vi "MultiSegmentSpectroscopy.vi"() -> ()   [LabVIEW 2019]
doc: "Performs a Bias Spectroscopy consisting of several user-definable segments.\n\n- Nanonis Programming Interface -"
uses:
  <userlib>/Nanonis Prog Interface V5/Nanonis Prog Interface.lvlib
panel:
  in  "Switch off Delay (s)":sgl min=0 max=100 format="%#_6p"
  in  "TipLift (m)":dbl format="%#_6p"
  out "SaveData":refnum<k4>
  in  "Save Data":bool
  out "Data":sgl[][](array[numeric])
  out "Index":u32[](array[numeric])
  out "UpdateGraphs":refnum<k4>
  out "RunSpec":refnum<k4>
  out "Change Params":refnum<k4>
  out "Sig_vs_Bias":cluster{sgl[], sgl[]}(graph)
  in  "Channel":u16(ring)
  out "Sig_vs_Ind":cluster{u32[], sgl[]}(graph)
  in  "Run Spectroscopy":bool
  out "Voltage Sequence":T1(graph)=[{"Data Points"=[0.0, 1.0, 2.0, 3.0, 4.0, 5.0, 6.0, 7.0, 8.0, 9.0, 10.0, 11.0, 12.0, 13.0, 14.0, 15.0, 16.0, 17.0, 18.0, 19.0, 20.0, 21.0, 22.0, 23.0, 24.0, 25.0, 26.0, 27.0, 28.0, 29.0, 30.0, 31.0, 32.0, 33.0, 34.0, 35.0, 36.0, 37.0, 38.0, 39.0, 40.0, 41.0, 42.0, 43.0, 44.0, 45.0, 46.0, 47.0, 48.0, 49.0], "Data Points"=[-1.0, -0.9836734693877551, -0.9673469387755103, -0.9510204081632653, -0.9346938775510204, -0.9183673469387755, -0.9020408163265305, -0.8857142857142857, -0.8693877551020408, -0.8530612244897959, -0.8367346938775511, -0.8204081632653061, -0.8040816326530612, -0.7877551020408163, -0.7714285714285714, -0.7551020408163265, -0.7387755102040816, -0.7224489795918367, -0.7061224489795919, -0.6897959183673469, -0.673469387755102, -0.6571428571428571, -0.6408163265306122, -0.6244897959183673, -0.6081632653061224, -0.5918367346938775, -0.5755102040816327, -0.5591836734693877, -0.5428571428571428, -0.5265306122448979, -0.510204081632653, -0.4938775510204081, -0.4775510204081632, -0.46122448979591835, -0.4448979591836735, -0.4285714285714285, -0.4122448979591836, -0.39591836734693875, -0.37959183673469377, -0.3632653061224489, -0.346938775510204, -0.33061224489795915, -0.3142857142857143, -0.2979591836734693, -0.2816326530612244, -0.26530612244897955, -0.24897959183673457, -0.2326530612244897, -0.21632653061224483, -0.19999999999999996]}, {"Data Points"=[50.0, 51.0, 52.0, 53.0, 54.0, 55.0, 56.0, 57.0, 58.0, 59.0, 60.0, 61.0, 62.0, 63.0, 64.0, 65.0, 66.0, 67.0, 68.0, 69.0, 70.0, 71.0, 72.0, 73.0, 74.0, 75.0, 76.0, 77.0, 78.0, 79.0, 80.0, 81.0, 82.0, 83.0, 84.0, 85.0, 86.0, 87.0, 88.0, 89.0, 90.0, 91.0, 92.0, 93.0, 94.0, 95.0, 96.0, 97.0, 98.0, 99.0, 100.0, 101.0, 102.0, 103.0, 104.0, 105.0, 106.0, 107.0, 108.0, 109.0, 110.0, 111.0, 112.0, 113.0, 114.0, 115.0, 116.0, 117.0, 118.0, 119.0, 120.0, 121.0, 122.0, 123.0, 124.0, 125.0, 126.0, 127.0, 128.0, 129.0, 130.0, 131.0, 132.0, 133.0, 134.0, 135.0, 136.0, 137.0, 138.0, 139.0, 140.0, 141.0, 142.0, 143.0, 144.0, 145.0, 146.0, 147.0, 148.0, 149.0, 150.0, 151.0, 152.0, 153.0, 154.0, 155.0, 156.0, 157.0, 158.0, 159.0, 160.0, 161.0, 162.0, 163.0, 164.0, 165.0, 166.0, 167.0, 168.0, 169.0, 170.0, 171.0, 172.0, 173.0, 174.0, 175.0, 176.0, 177.0, 178.0, 179.0, 180.0, 181.0, 182.0, 183.0, 184.0, 185.0, 186.0, 187.0, 188.0, 189.0, 190.0, 191.0, 192.0, 193.0, 194.0, 195.0, 196.0, 197.0, 198.0, 199.0, 200.0, 201.0, 202.0, 203.0, 204.0, 205.0, 206.0, 207.0, 208.0, 209.0, 210.0, 211.0, 212.0, 213.0, 214.0, 215.0, 216.0, 217.0, 218.0, 219.0, 220.0, 221.0, 222.0, 223.0, 224.0, 225.0, 226.0, 227.0, 228.0, 229.0, 230.0, 231.0, 232.0, 233.0, 234.0, 235.0, 236.0, 237.0, 238.0, 239.0, 240.0, 241.0, 242.0, 243.0, 244.0, 245.0, 246.0, 247.0, 248.0, 249.0, 250.0, 251.0, 252.0, 253.0, 254.0, 255.0, 256.0, 257.0, 258.0, 259.0, 260.0, 261.0, 262.0, 263.0, 264.0, 265.0, 266.0, 267.0, 268.0, 269.0, 270.0, 271.0, 272.0, 273.0, 274.0, 275.0, 276.0, 277.0, 278.0, 279.0, 280.0, 281.0, 282.0, 283.0, 284.0, 285.0, 286.0, 287.0, 288.0, 289.0, 290.0, 291.0, 292.0, 293.0, 294.0, 295.0, 296.0, 297.0, 298.0, 299.0, 300.0, 301.0, 302.0, 303.0, 304.0, 305.0, 306.0, 307.0, 308.0, 309.0, 310.0, 311.0, 312.0, 313.0, 314.0, 315.0, 316.0, 317.0, 318.0, 319.0, 320.0, 321.0, 322.0, 323.0, 324.0, 325.0, 326.0, 327.0, 328.0, 329.0, 330.0, 331.0, 332.0, 333.0, 334.0, 335.0, 336.0, 337.0, 338.0, 339.0, 340.0, 341.0, 342.0, 343.0, 344.0, 345.0, 346.0, 347.0, 348.0, 349.0, 350.0, 351.0, 352.0, 353.0, 354.0, 355.0, 356.0, 357.0, 358.0, 359.0, 360.0, 361.0, 362.0, 363.0, 364.0, 365.0, 366.0, 367.0, 368.0, 369.0, 370.0, 371.0, 372.0, 373.0, 374.0, 375.0, 376.0, 377.0, 378.0, 379.0, 380.0, 381.0, 382.0, 383.0, 384.0, 385.0, 386.0, 387.0, 388.0, 389.0, 390.0, 391.0, 392.0, 393.0, 394.0, 395.0, 396.0, 397.0, 398.0, 399.0, 400.0, 401.0, 402.0, 403.0, 404.0, 405.0, 406.0, 407.0, 408.0, 409.0, 410.0, 411.0, 412.0, 413.0, 414.0, 415.0, 416.0, 417.0, 418.0, 419.0, 420.0, 421.0, 422.0, 423.0, 424.0, 425.0, 426.0, 427.0, 428.0, 429.0, 430.0, 431.0, 432.0, 433.0, 434.0, 435.0, 436.0, 437.0, 438.0, 439.0, 440.0, 441.0, 442.0, 443.0, 444.0, 445.0, 446.0, 447.0, 448.0, 449.0], "Data Points"=[-0.2, -0.19899749373433584, -0.1979949874686717, -0.19699248120300752, -0.19598997493734338, -0.1949874686716792, -0.19398496240601504, -0.1929824561403509, -0.19197994987468672, -0.19097744360902258, -0.1899749373433584, -0.18897243107769424, -0.1879699248120301, -0.18696741854636592, -0.18596491228070178, -0.1849624060150376, -0.18395989974937343, -0.1829573934837093, -0.18195488721804512, -0.18095238095238098, -0.1799498746867168, -0.17894736842105263, -0.1779448621553885, -0.17694235588972432, -0.17593984962406017, -0.174937343358396, -0.17393483709273183, -0.1729323308270677, -0.17192982456140352, -0.17092731829573937, -0.1699248120300752, -0.16892230576441103, -0.16791979949874689, -0.16691729323308271, -0.16591478696741857, -0.1649122807017544, -0.16390977443609023, -0.16290726817042608, -0.1619047619047619, -0.16090225563909777, -0.1598997493734336, -0.15889724310776943, -0.15789473684210528, -0.1568922305764411, -0.15588972431077697, -0.1548872180451128, -0.15388471177944862, -0.15288220551378448, -0.1518796992481203, -0.15087719298245617, -0.149874686716792, -0.14887218045112782, -0.14786967418546368, -0.1468671679197995, -0.14586466165413536, -0.1448621553884712, -0.14385964912280702, -0.14285714285714288, -0.1418546365914787, -0.14085213032581456, -0.1398496240601504, -0.13884711779448622, -0.13784461152882208, -0.1368421052631579, -0.13583959899749376, -0.1348370927318296, -0.13383458646616542, -0.13283208020050125, -0.1318295739348371, -0.13082706766917296, -0.1298245614035088, -0.12882205513784462, -0.12781954887218044, -0.1268170426065163, -0.12581453634085216, -0.12481203007518799, -0.12380952380952383, -0.12280701754385966, -0.1218045112781955, -0.12080200501253134, -0.11979949874686718, -0.11879699248120303, -0.11779448621553885, -0.1167919799498747, -0.11578947368421054, -0.11478696741854638, -0.11378446115288222, -0.11278195488721805, -0.1117794486215539, -0.11077694235588974, -0.10977443609022558, -0.10877192982456142, -0.10776942355889725, -0.1067669172932331, -0.10576441102756894, -0.10476190476190478, -0.1037593984962406, -0.10275689223057645, -0.10175438596491229, -0.10075187969924813, -0.09974937343358398, -0.0987468671679198, -0.09774436090225565, -0.09674185463659149, -0.09573934837092733, -0.09473684210526317, -0.093734335839599, -0.09273182957393485, -0.09172932330827069, -0.09072681704260653, -0.08972431077694237, -0.0887218045112782, -0.08771929824561404, -0.08671679197994989, -0.08571428571428573, -0.08471177944862157, -0.0837092731829574, -0.08270676691729324, -0.08170426065162908, -0.08070175438596493, -0.07969924812030077, -0.0786967418546366, -0.07769423558897244, -0.07669172932330828, -0.07568922305764413, -0.07468671679197997, -0.0736842105263158, -0.07268170426065165, -0.07167919799498748, -0.07067669172932331, -0.06967418546365917, -0.068671679197995, -0.06766917293233085, -0.06666666666666668, -0.06566416040100251, -0.06466165413533836, -0.06365914786967419, -0.06265664160401005, -0.06165413533834588, -0.060651629072681706, -0.05964912280701756, -0.05864661654135339, -0.05764411027568925, -0.056641604010025076, -0.055639097744360905, -0.05463659147869676, -0.05363408521303259, -0.052631578947368446, -0.051629072681704274, -0.0506265664160401, -0.04962406015037596, -0.04862155388471179, -0.047619047619047644, -0.04661654135338347, -0.0456140350877193, -0.04461152882205516, -0.043609022556390986, -0.04260651629072684, -0.04160401002506267, -0.0406015037593985, -0.039598997493734356, -0.038596491228070184, -0.03759398496240604, -0.03659147869674187, -0.0355889724310777, -0.034586466165413554, -0.03358395989974938, -0.03258145363408524, -0.03157894736842107, -0.030576441102756896, -0.029573934837092752, -0.02857142857142858, -0.027568922305764437, -0.026566416040100266, -0.025563909774436094, -0.02456140350877195, -0.02355889724310778, -0.022556390977443636, -0.021553884711779464, -0.020551378446115293, -0.01954887218045115, -0.018546365914786977, -0.017543859649122834, -0.016541353383458662, -0.015538847117794491, -0.014536340852130347, -0.013533834586466176, -0.012531328320802032, -0.01152882205513786, -0.01052631578947369, -0.009523809523809545, -0.008521303258145374, -0.007518796992481203, -0.006516290726817059, -0.0055137844611528875, -0.004511278195488744, -0.0035087719298245723, -0.002506265664160401, -0.0015037593984962572, -0.0005012531328320857, 0.000501253132832058, 0.0015037593984962294, 0.002506265664160401, 0.0035087719298245446, 0.004511278195488716, 0.00551378446115286, 0.006516290726817031, 0.007518796992481203, 0.008521303258145346, 0.009523809523809518, 0.010526315789473661, 0.011528822055137833, 0.012531328320802004, 0.013533834586466148, 0.01453634085213032, 0.015538847117794463, 0.016541353383458635, 0.017543859649122806, 0.01854636591478695, 0.01954887218045112, 0.020551378446115265, 0.021553884711779436, 0.022556390977443608, 0.02355889724310775, 0.024561403508771923, 0.025563909774436067, 0.026566416040100238, 0.02756892230576441, 0.028571428571428553, 0.029573934837092725, 0.03057644110275687, 0.03157894736842104, 0.03258145363408521, 0.033583959899749355, 0.034586466165413526, 0.03558897243107767, 0.03659147869674184, 0.03759398496240601, 0.03859649122807016, 0.03959899749373433, 0.04060150375939847, 0.04160401002506264, 0.042606516290726815, 0.04360902255639096, 0.04461152882205513, 0.045614035087719274, 0.046616541353383445, 0.047619047619047616, 0.04862155388471176, 0.04962406015037593, 0.050626566416040075, 0.05162907268170425, 0.05263157894736842, 0.05363408521303259, 0.054636591478696706, 0.05563909774436088, 0.05664160401002505, 0.05764411027568922, 0.05864661654135339, 0.05964912280701751, 0.06065162907268168, 0.06165413533834585, 0.06265664160401002, 0.06365914786967419, 0.06466165413533831, 0.06566416040100248, 0.06666666666666665, 0.06766917293233082, 0.068671679197995, 0.06967418546365911, 0.07067669172932328, 0.07167919799498745, 0.07268170426065163, 0.0736842105263158, 0.07468671679197991, 0.07568922305764408, 0.07669172932330826, 0.07769423558897243, 0.0786967418546366, 0.07969924812030071, 0.08070175438596489, 0.08170426065162906, 0.08270676691729323, 0.0837092731829574, 0.08471177944862152, 0.08571428571428569, 0.08671679197994986, 0.08771929824561403, 0.0887218045112782, 0.08972431077694232, 0.09072681704260649, 0.09172932330827066, 0.09273182957393483, 0.093734335839599, 0.09473684210526312, 0.09573934837092729, 0.09674185463659146, 0.09774436090225563, 0.0987468671679198, 0.09974937343358392, 0.10075187969924809, 0.10175438596491226, 0.10275689223057644, 0.1037593984962406, 0.10476190476190472, 0.1057644110275689, 0.10676691729323307, 0.10776942355889724, 0.10877192982456141, 0.10977443609022552, 0.1107769423558897, 0.11177944862155387, 0.11278195488721804, 0.11378446115288221, 0.11478696741854633, 0.1157894736842105, 0.11679197994987467, 0.11779448621553884, 0.11879699248120301, 0.11979949874686713, 0.1208020050125313, 0.12180451127819547, 0.12280701754385964, 0.12380952380952381, 0.12481203007518793, 0.1258145363408521, 0.12681704260651627, 0.12781954887218044, 0.12882205513784462, 0.12982456140350873, 0.1308270676691729, 0.13182957393483707, 0.13283208020050125, 0.13383458646616542, 0.13483709273182953, 0.1358395989974937, 0.13684210526315788, 0.13784461152882205, 0.13884711779448622, 0.13984962406015033, 0.1408521303258145, 0.14185463659147868, 0.14285714285714285, 0.14385964912280702, 0.14486215538847114, 0.1458646616541353, 0.14686716791979948, 0.14786967418546365, 0.14887218045112782, 0.14987468671679194, 0.1508771929824561, 0.15187969924812028, 0.15288220551378445, 0.15388471177944862, 0.15488721804511274, 0.1558897243107769, 0.15689223057644108, 0.15789473684210525, 0.15889724310776943, 0.15989974937343354, 0.1609022556390977, 0.16190476190476188, 0.16290726817042606, 0.16390977443609023, 0.16491228070175434, 0.16591478696741851, 0.1669172932330827, 0.16791979949874686, 0.16892230576441103, 0.16992481203007515, 0.17092731829573932, 0.1719298245614035, 0.17293233082706766, 0.17393483709273183, 0.17493734335839595, 0.17593984962406012, 0.1769423558897243, 0.17794486215538846, 0.17894736842105263, 0.17994987468671675, 0.18095238095238092, 0.1819548872180451, 0.18295739348370926, 0.18395989974937343, 0.1849624060150376, 0.18596491228070172, 0.1869674185463659, 0.18796992481203006, 0.18897243107769424, 0.1899749373433584, 0.19097744360902252, 0.1919799498746867, 0.19298245614035087, 0.19398496240601504, 0.1949874686716792, 0.19598997493734333, 0.1969924812030075, 0.19799498746867167, 0.19899749373433584, 0.2]}, ...(3 in all)]
  out "AllQuit":bool
  in  "stop":bool
  in  "Autosave Data":enum16{"no change", "on", "off"}(ring)
  in  "Parameters":T2(array[cluster])=[{"Start"=-1.0, "Stop"=-0.2, "# Points"=50}, {"Start"=-0.2, "Stop"=0.2, "# Points"=400}, {"Start"=0.2, "Stop"=1.0, "# Points"=50}] {"# Points" min=2; "Stop" format="%1_3p"; "Start" format="%1_3p"}
  # "Temporary Variables"
  # "Z-Controller"
  # "Note:\nTo insert or remove a \nsegment right-click in \nthe parameter section"
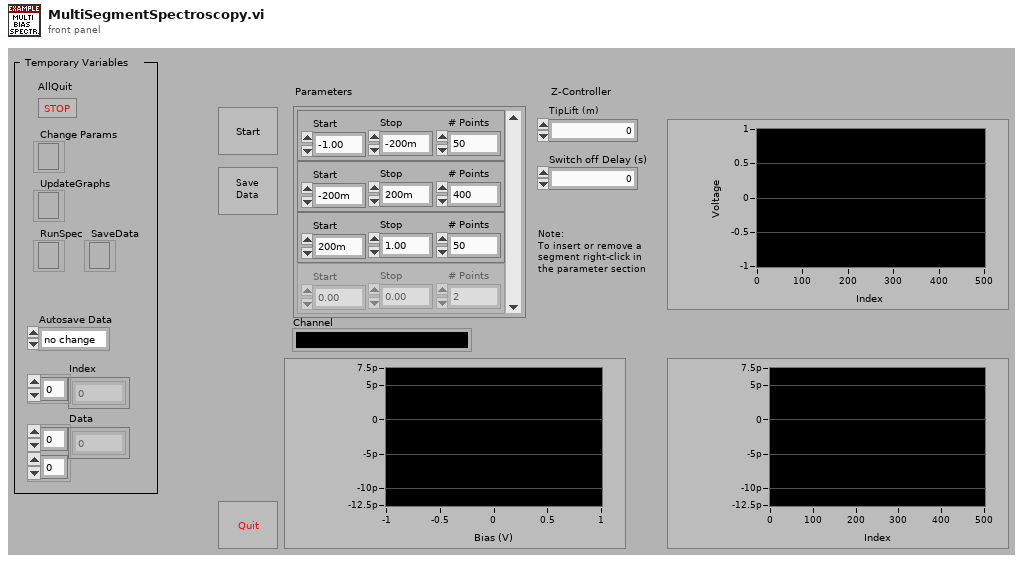
[diagram p1: front panel]
types:
  T1 = cluster{"Data Points":dbl[], "Data Points":dbl[]}[]
  T2 = cluster{"Start":dbl, "Stop":dbl, "# Points":i32}[]
  T3 = cluster{"Data Points":dbl[], "Data Points":dbl[]}
  T4 = cluster{"End settling time (s)":sgl, "Z control time (s)":sgl}
  T5 = cluster{"Z averaging time (s)":sgl, "Z offset (m)":sgl, "Initial settling time (s)":sgl}
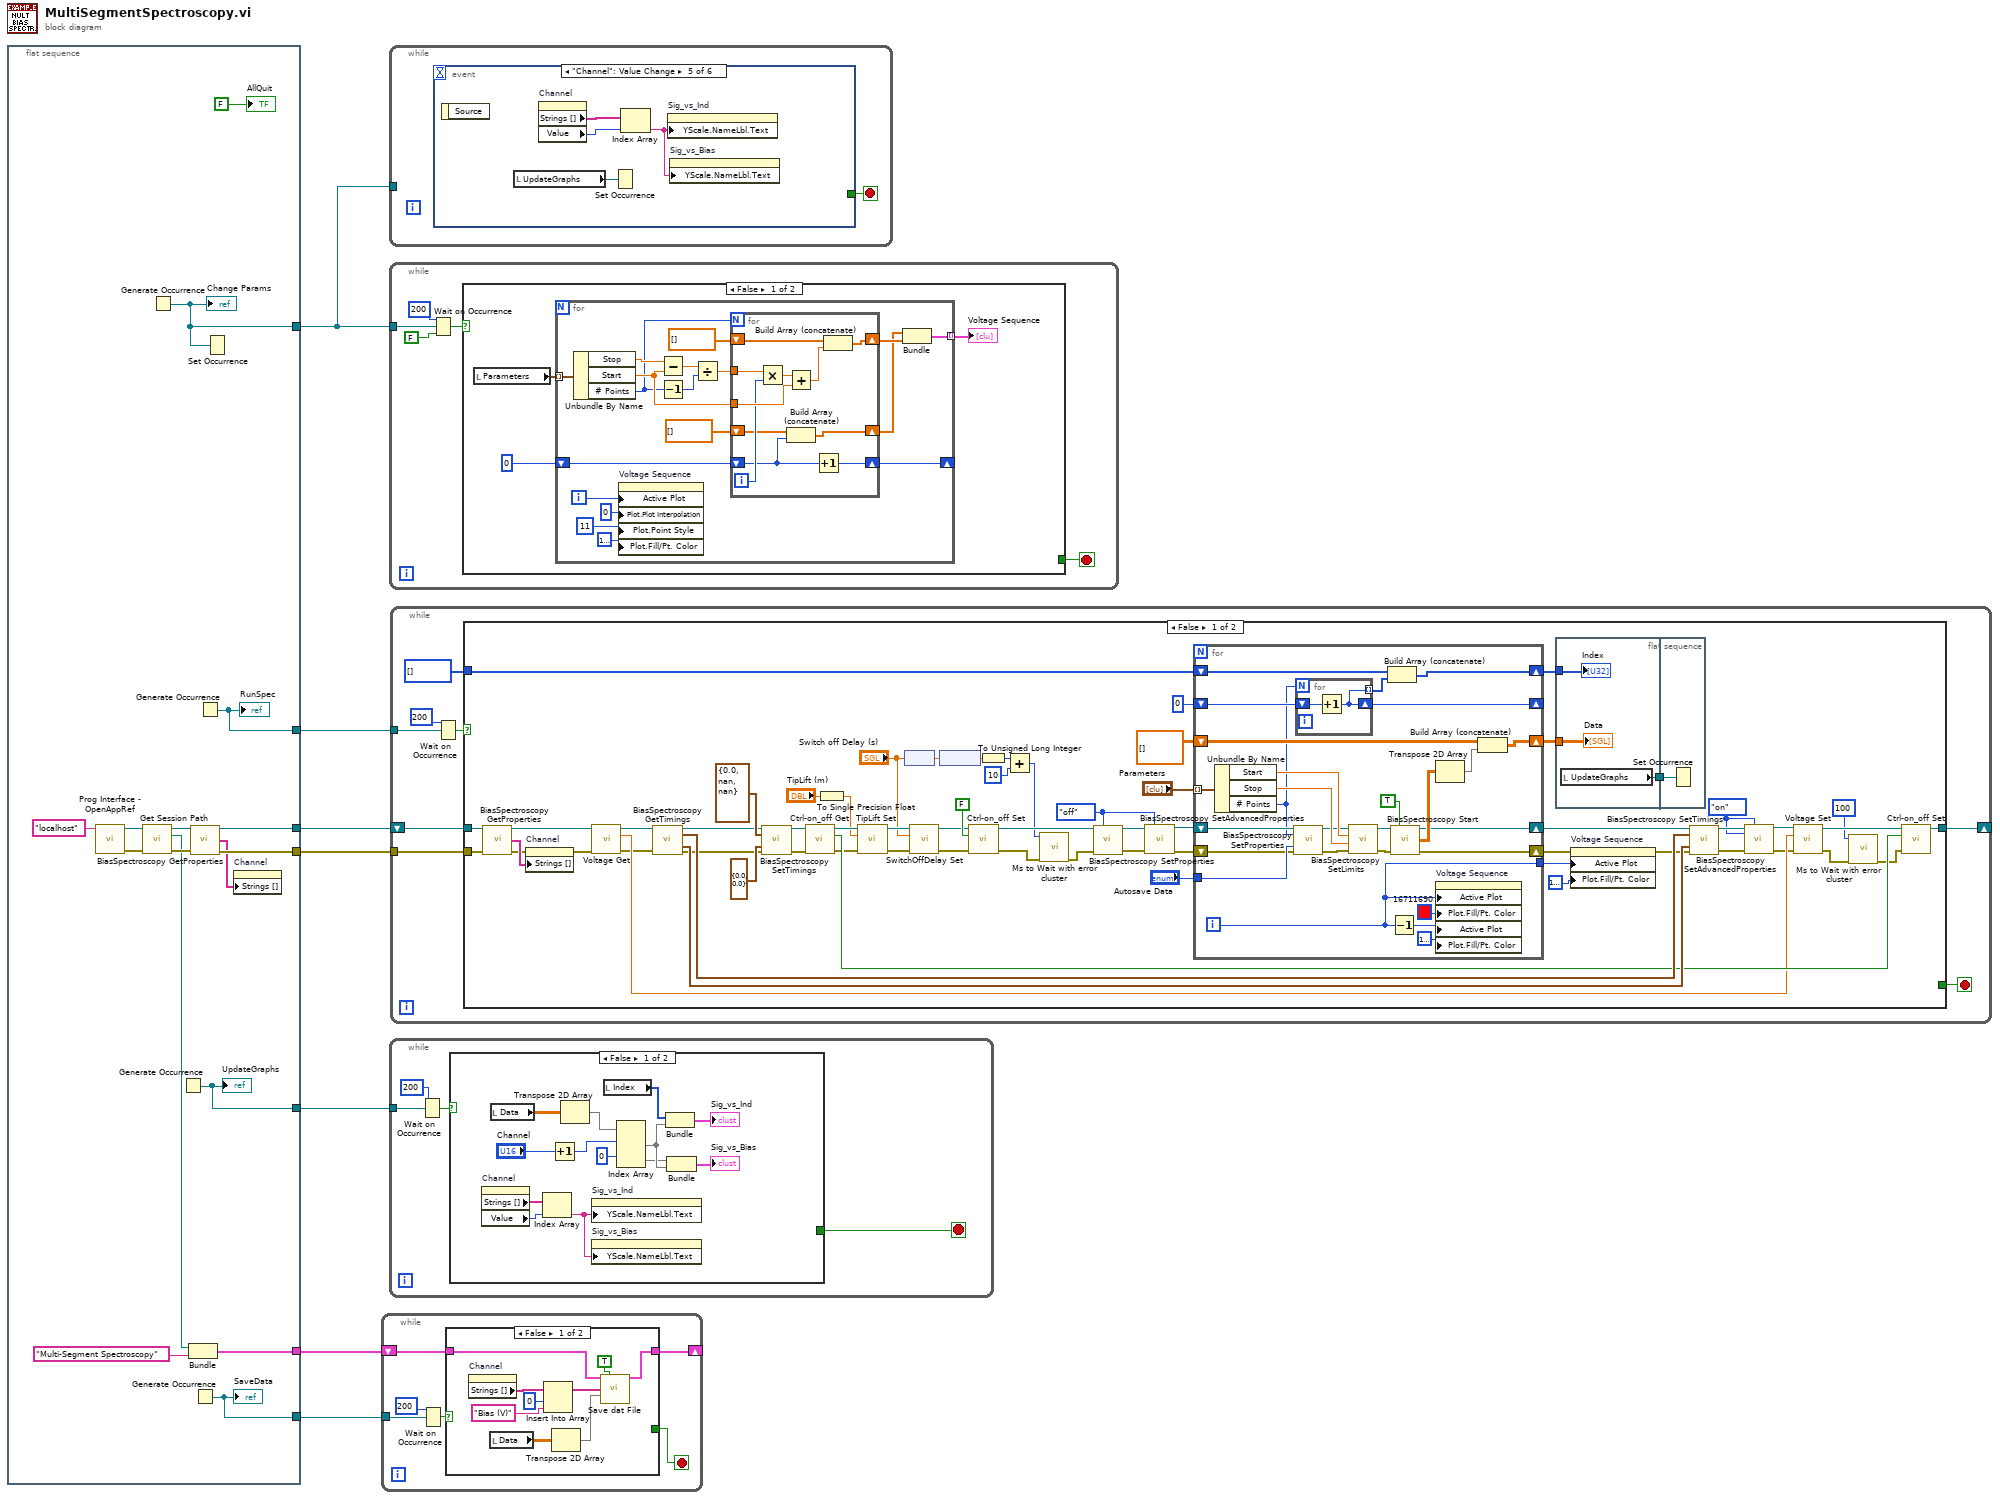
[diagram p0: block diagram]
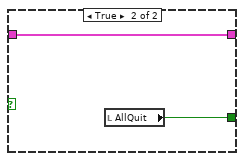
[diagram p2: hidden frame]
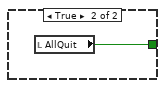
[diagram p3: hidden frame]
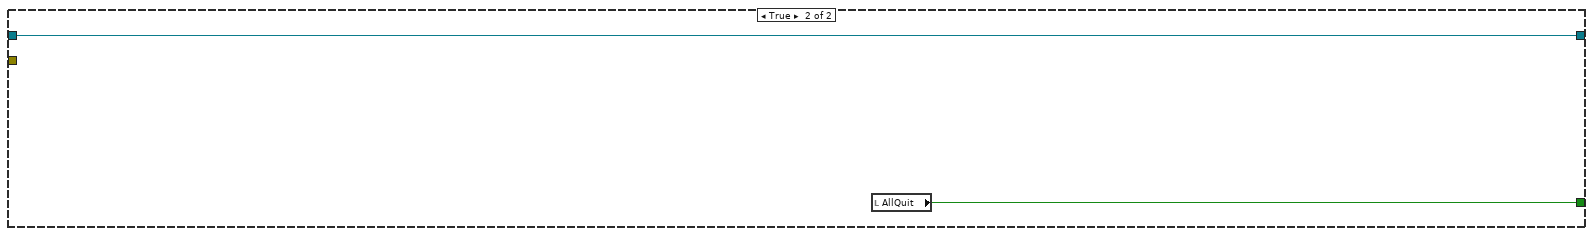
[diagram p4: hidden frame]
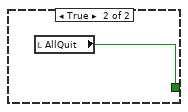
[diagram p5: hidden frame]
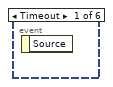
[diagram p6: hidden frame]
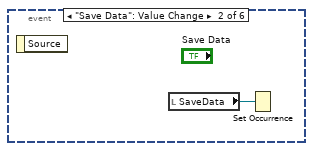
[diagram p7: hidden frame]
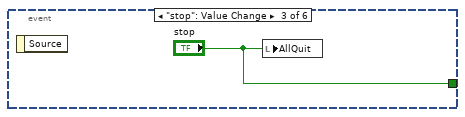
[diagram p8: hidden frame]
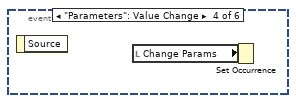
[diagram p9: hidden frame]
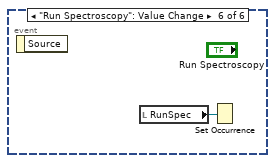
[diagram p10: hidden frame]
diagram:
  n1 = flat-sequence {
    tunnel: [w19] -> w7
    tunnel: [w20] -> w5
    tunnel: [w17] -> w6
    tunnel: [w21] -> w4
    tunnel: [w18] -> w3
    tunnel: [w16] -> w2
    tunnel: [w8] -> w1
    frame #0 {
      n2 = call <userlib>:"Prog Interface - OpenAppRef.vi"("Machine name (local machine IP)"="localhost" ("Machine name (localhost)")) -> ("Error out"=w11:errorcluster, "Application reference"=w14:refnum<vi>)  [unwired: 5 in]
      n3 = call <userlib>:"Get Session Path.vi"("error in (no error)"=w11, "Application ref in"=w14) -> ("error out"=w12:errorcluster, "Session path"=w9:path, "Application ref out"=w13:refnum<vi>)  [unwired: 7 in]
      n4 = Generate Occurrence() -> (w20:refnum<k4>)
      "Change Params" <- w20
      n5 = Generate Occurrence() -> (w21:refnum<k4>)
      "UpdateGraphs" <- w21
      n6 = Bundle("Session path"=w9, "Basename"="Multi-Segment Spectroscopy") -> (w8:cluster{"Session path":path, "Basename":string})  [unwired: 1 in]
      n7 = call <userlib>:"BiasSpectroscopy GetProperties.vi"("Application ref in"=w13, "Error in (no error)"=w12) -> ("Application ref out"=w16:refnum<vi>, "Channels"=w15:string[], "Error out"=w19:errorcluster)  [unwired: 6 in, 5 out]
      n8 = Generate Occurrence() -> (w18:refnum<k4>)
      "SaveData" <- w18
      n9 = Generate Occurrence() -> (w17:refnum<k4>)
      "RunSpec" <- w17
      n10 = Set Occurrence(w20) -> ()
      n11 = property on="Channel" class="Ring (strict)"("Strings []"=w15) -> ()  [unwired: 2 in, 2 out]
      "AllQuit" <- FALSE ("AllQuit")
    }
  }
  n12 = while {
    tunnel: w3 -> [w27]
    shift-right: [w24] -> _
    shift-left: w1 -> [w25]
    stop <- w28 stop-if-true
    n13 = Wait on Occurrence(2:w27, 3:200 ("ms timeout (-1)")) -> (0:w29:bool)  [unwired: 1 in]
    n14 = case shown="False" w29 {
      tunnel: [_ w40] -> w28
      tunnel: w25 -> [w31 w39]
      tunnel: [w30 w39] -> w24
      frame False {
        n15 = property on="Channel" class="Ring (strict)"() -> ("Strings []"=w37:string[])  [unwired: 2 in, 2 out]
        n16 = local read "Data"() -> (w34:sgl[][])
        n17 = Insert Into Array(array=w37, index=0, new element="Bias (V)") -> (w35:string[])
        n18 = Transpose 2D Array(2D array=w34) -> (transposed array=w33:sgl[][])
        n19 = call <userlib>:"Save dat File.vi"("Filename control"=w31, "Show save dialog (T)"=TRUE, "Channels names"=w35, "Data"=w33) -> ("Filename control out"=w30:cluster{"Path":path, "Basename":string})  [unwired: 8 in, 3 out]
      }
      frame True {
        n20 = local read "AllQuit"() -> (w40:bool)
      }
    }
  }
  n21 = while {
    tunnel: w5 -> [_]
    stop <- w41 stop-if-true
    n22 = event shown="[4] \"Channel\": Value Change" {
      selector: _ -> [_ _ _ _ _ _]
      dyn-events: _ -> [_ _ _ _ _ _]
      timeout: _ -> [_ _ _ _ _ _]
      tunnel: [_ _ "stop" _ _ _] -> w41
      event Timeout {
        n23 = event-data() -> ()  [unwired: 1 in, 1 out]
      }
      event "Save Data": Value Change {
        n24 = event-data() -> ()  [unwired: 1 in, 1 out]
        n25 = local read "SaveData"() -> (w42:refnum<k4>)
        n26 = Set Occurrence(w42) -> ()
      }
      event "stop": Value Change {
        n27 = event-data() -> ()  [unwired: 1 in, 1 out]
        n28 = local write "AllQuit"("stop") -> ()
      }
      event "Parameters": Value Change {
        n29 = event-data() -> ()  [unwired: 1 in, 1 out]
        n30 = local read "Change Params"() -> (w44:refnum<k4>)
        n31 = Set Occurrence(w44) -> ()
      }
      event "Channel": Value Change {
        n32 = event-data() -> ()  [unwired: 1 in, 1 out]
        n33 = local read "UpdateGraphs"() -> (w46:refnum<k4>)
        n34 = property on="Channel" class="Ring (strict)"() -> ("Strings []"=w48:string[], "Value"=w45:u16)  [unwired: 2 in, 2 out]
        n35 = Set Occurrence(w46) -> ()
        n36 = Index Array(array=w48, index=w45) -> (element=w47:string)
        n37 = property on="Sig_vs_Ind" class="XYGraph (strict)"("YScale.NameLbl.Text"=w47) -> ()  [unwired: 2 in, 2 out]
        n38 = property on="Sig_vs_Bias" class="XYGraph (strict)"("YScale.NameLbl.Text"=w47) -> ()  [unwired: 2 in, 2 out]
      }
      event "Run Spectroscopy": Value Change {
        n39 = event-data() -> ()  [unwired: 1 in, 1 out]
        n40 = local read "RunSpec"() -> (w49:refnum<k4>)
        n41 = Set Occurrence(w49) -> ()
      }
    }
  }
  n42 = while {
    tunnel: w5 -> [w54]
    stop <- w51 stop-if-true
    n43 = Wait on Occurrence(1:FALSE ("ignore previous (T)"), 2:w54, 3:200 ("ms timeout (-1)")) -> (0:w52:bool)
    n44 = case shown="False" w52 {
      tunnel: [_ w87] -> w51
      frame False {
        n45 = local read "Parameters"() -> (w55:T2)
        n46 = for {
          shift-right: [w68] -> _
          shift-left: u16 0 ("# Points") -> [w69]
          tunnel: [w66] -> w56 mode=indexing
          tunnel: w55 -> [w58] mode=indexing
          i -> [w63]
          n47 = Unbundle By Name(w58) -> ("Stop"=w75:dbl, "Start"=w74:dbl, "# Points"=w70:i32)
          n48 = property on="Voltage Sequence" class="XYGraph (strict)"("Active Plot"=w63, "Plot.Plot Interpolation"=u8 0 ("Plot.Line Style"), "Plot.Point Style"=u8 11 ("Plot.Line Style"), "Plot.Fill/Pt. Color"=u32 16777226) -> ()  [unwired: 2 in, 2 out]
          n49 = Subtract(x=w75, y=w74) -> (x-y=w73:dbl)
          n50 = Decrement(x=w70) -> (x-1=w71:i32)
          n51 = Divide(x=w73, y=w71) -> (x/y=w72:dbl)
          n52 = for {
            N: w70 -> [_]
            tunnel: w72 -> [w86]
            tunnel: w74 -> [w84]
            shift-right: [w79] -> w67
            shift-left: sgl[] [] ("Data Points") -> [w80]
            shift-right: [w81] -> w59
            shift-left: dbl[] [] ("Data Points") -> [w82]
            shift-right: [w76] -> w68
            shift-left: w69 -> [w77]
            i -> [w83]
            n53 = Multiply(x=w86, y=w83) -> (x*y=w85:dbl)
            n54 = Add(x=w85, y=w84) -> (x+y=w78:dbl)
            n55 = Build Array (concatenate)(w82, w77) -> (w81:dbl[])
            n56 = Increment(x=w77) -> (x+1=w76:u16)
            n57 = Build Array (concatenate)(w80, w78) -> (w79:dbl[])
          }
          n58 = Bundle("Data Points"=w59, "Data Points"=w67) -> (w66:T3)  [unwired: 1 in]
        }
        "Voltage Sequence" <- w56
      }
      frame True {
        n59 = local read "AllQuit"() -> (w87:bool)
      }
    }
  }
  n60 = while {
    tunnel: w4 -> [w91]
    stop <- w88 stop-if-true
    n61 = Wait on Occurrence(2:w91, 3:200 ("ms timeout (-1)")) -> (0:w89:bool)  [unwired: 1 in]
    n62 = case shown="False" w89 {
      tunnel: [_ w105] -> w88
      frame False {
        n63 = property on="Channel" class="Ring (strict)"() -> ("Strings []"=w94:string[], "Value"=w93:u16)  [unwired: 2 in, 2 out]
        n64 = local read "Data"() -> (w100:sgl[][])
        n65 = Index Array(array=w94, index=w93) -> (element=w92:string)
        n66 = Increment(x="Channel") -> (x+1=w98:u16)
        n67 = Transpose 2D Array(2D array=w100) -> (transposed array=w99:sgl[][])
        n68 = property on="Sig_vs_Ind" class="XYGraph (strict)"("YScale.NameLbl.Text"=w92) -> ()  [unwired: 2 in, 2 out]
        n69 = property on="Sig_vs_Bias" class="XYGraph (strict)"("YScale.NameLbl.Text"=w92) -> ()  [unwired: 2 in, 2 out]
        n70 = local read "Index"() -> (w104:u32[])
        n71 = Index Array(array=w99, index (row) #1=w98, index (row) #2=0 ("index (row)")) -> (element #1=w103:sgl[], element #2=w101:sgl[])  [unwired: 2 in]
        n72 = Bundle("Index"=w104, w103) -> (→"Sig_vs_Ind":cluster{"Index":u32[], sgl[]})  [unwired: 1 in]
        n73 = Bundle(w101, w103) -> (→"Sig_vs_Bias":cluster{sgl[], sgl[]})  [unwired: 1 in]
      }
      frame True {
        n74 = local read "AllQuit"() -> (w105:bool)
      }
    }
  }
  n75 = while {
    tunnel: w7 -> [w113]
    tunnel: w6 -> [w112]
    shift-right: [w106] -> _
    shift-left: w2 -> [w107]
    stop <- w109 stop-if-true
    n76 = Wait on Occurrence(2:w112, 3:200 ("ms timeout (-1)")) -> (0:w110:bool)  [unwired: 1 in]
    n77 = case shown="False" w110 {
      tunnel: w113 -> [w158 _]
      tunnel: [_ w212] -> w109
      tunnel: u32[] [] ("Data Points") -> [w174 _]
      tunnel: w107 -> [w159 w211]
      tunnel: [w145 w211] -> w106
      frame False {
        w114 = enum16{"no change", "on", "off"}."on" ("Reset Bias (no change)")
        w119 = enum16{"no change", "on", "off"}."off" ("Reset Bias (no change)")
        n78 = call <userlib>:"BiasSpectroscopy GetProperties.vi"("Application ref in"=w159, "Error in (no error)"=w158) -> ("Application ref out"=w156:refnum<vi>, "Channels"=w167:string[], "Error out"=w163:errorcluster)  [unwired: 6 in, 5 out]
        n79 = property on="Channel" class="Ring (strict)"(error in=w163, "Strings []"=w167) -> (error out=w157:errorcluster)  [unwired: 1 in, 1 out]
        n80 = call <userlib>:"Voltage Get.vi"("error in (no error)"=w157, "Application ref in"=w156) -> ("error out"=w149:errorcluster, "Bias (V)"=w155:sgl, "Application ref out"=w152:refnum<vi>)  [unwired: 7 in]
        n81 = call <userlib>:"BiasSpectroscopy GetTimings.vi"("Application ref in"=w152, "Error in (no error)"=w149) -> ("Application ref out"=w151:refnum<vi>, "Initialization"=w165:T5, "End of Sweep"=w164:T4, "Error out"=w148:errorcluster)  [unwired: 9 in, 1 out]
        n82 = call <userlib>:"BiasSpectroscopy SetTimings.vi"("Application ref in"=w151, "Initialization (NaN)"=T5 {"Z averaging time (s)"=0.0, "Z offset (m)"=nan, "Initial settling time (s)"=nan}, "End of Sweep (NaN)"=T4 {"End settling time (s)"=0.0, "Z control time (s)"=0.0}, "Error in (no error)"=w148) -> ("Application ref out"=w150:refnum<vi>, "Error out"=w147:errorcluster)  [unwired: 10 in]
        n83 = call <userlib>:"Ctrl-on_off Get.vi"("error in (no error)"=w147, "Application ref in"=w150) -> ("error out"=w138:errorcluster, "Z-Controller on/off status"=w160:bool, "Application ref out"=w139:refnum<vi>)  [unwired: 7 in]
        n84 = To Single Precision Float(number="TipLift (m)") -> (single precision float=w133:sgl)
        n85 = call <userlib>:"TipLift Set.vi"("error in (no error)"=w138, "TipLift (m)"=w133, "Application ref in"=w139) -> ("error out"=w135:errorcluster, "Application ref out"=w137:refnum<vi>)  [unwired: 7 in]
        n86 = node("Switch off Delay (s)") -> (w131:sgl[unit])
        n87 = call <userlib>:"SwitchOffDelay Set.vi"("error in (no error)"=w135, "Switch off Delay (s)"="Switch off Delay (s)", "Application ref in"=w137) -> ("error out"=w126:errorcluster, "Application ref out"=w136:refnum<vi>)  [unwired: 7 in]
        n88 = node(w131) -> (w130:sgl)
        n89 = call <userlib>:"Ctrl-on_off Set.vi"("error in (no error)"=w126, "Z Controller ON/OFF"=FALSE, "Application ref in"=w136) -> ("error out"=w125:errorcluster, "Application ref out"=w144:refnum<vi>)  [unwired: 7 in]
        n90 = To Unsigned Long Integer(number=w130) -> (unsigned 32bit integer=w129:u32)
        n91 = Add(x=w129, y=u32 10) -> (x+y=w128:u32)
        n92 = call <userlib>:"Ms to Wait with error cluster.vi"("error in (no error)"=w125, "milliseconds to wait"=w128) -> ("error out"=w124:errorcluster)  [unwired: 4 in, 1 out]
        n93 = call <userlib>:"BiasSpectroscopy SetProperties.vi"("Application ref in"=w144, "Backward sweep (no change)"=w119, "Error in (no error)"=w124) -> ("Application ref out"=w120:refnum<vi>, "Error out"=w121:errorcluster)  [unwired: 11 in]
        n94 = call <userlib>:"BiasSpectroscopy SetAdvancedProperties.vi"("Application ref in"=w120, "Reset Bias (no change)"=w119, "Error in (no error)"=w121) -> ("Application ref out"=w123:refnum<vi>, "Error out"=w122:errorcluster)  [unwired: 11 in]
        n95 = for {
          tunnel: "Autosave Data" -> [w207]
          shift-right: [w202] -> w169
          shift-left: sgl[][] [] ("Data") -> [w203]
          tunnel: "Parameters" -> [w201] mode=indexing
          shift-right: [w195] -> w170
          shift-left: w174 -> [w200]
          shift-right: [w198] -> _
          shift-left: u32 0 -> [w199]
          tunnel: [w184] -> w172
          shift-right: [w188] -> w154
          shift-left: w123 -> [w193]
          shift-right: [w185] -> w166
          shift-left: w122 -> [w194]
          i -> [w184]
          n96 = Unbundle By Name(w201) -> ("Start"=w191:dbl, "Stop"=w192:dbl, "# Points"=w186:i32)
          n97 = call <userlib>:"BiasSpectroscopy SetProperties.vi"("Application ref in"=w193, "Number of points (0=no change)"=w186, "Autosave (no change)"=w207, "Error in (no error)"=w194) -> ("Application ref out"=w190:refnum<vi>, "Error out"=w206:errorcluster)  [unwired: 10 in]
          n98 = for {
            N: w186 -> [_]
            tunnel: [w210] -> w197 mode=indexing
            shift-right: [w210] -> w198
            shift-left: w199 -> [w209]
            n99 = Increment(x=w209) -> (x+1=w210:u32)
          }
          n100 = call <userlib>:"BiasSpectroscopy SetLimits.vi"("Error in (no error)"=w206, "End value (V)"=w192, "Start value (V)"=w191, "Application ref in"=w190) -> ("Error out"=w208:errorcluster, "Application ref out"=w189:refnum<vi>)  [unwired: 4 in]
          n101 = Build Array (concatenate)(w200, w197) -> (w195:u32[])
          n102 = Decrement(x=w184) -> (x-1=w183:i32)
          n103 = call <userlib>:"BiasSpectroscopy Start.vi"("Application ref in"=w189, "Get data (F)"=TRUE, "Error in (no error)"=w208) -> ("Application ref out"=w188:refnum<vi>, "Data"=w205:sgl[][], "Error out"=w185:errorcluster)  [unwired: 8 in, 2 out]
          n104 = Transpose 2D Array(2D array=w205) -> (transposed array=w204:sgl[][])
          n105 = property on="Voltage Sequence" class="XYGraph (strict)"("Active Plot"=w184, "Plot.Fill/Pt. Color"=u32 16711690, "Active Plot"=w183, "Plot.Fill/Pt. Color"=u32 16777226) -> ()  [unwired: 2 in, 2 out]
          n106 = Build Array (concatenate)(w203, w204) -> (w202:sgl[][])
        }
        n107 = flat-sequence {
          tunnel: w170 -> [w180]
          tunnel: w169 -> [w179]
          tunnel: [w178] -> w168
          tunnel: w168 -> [w181]
          frame #0 {
            n108 = local read "UpdateGraphs"() -> (w178:refnum<k4>)
            "Index" <- w180
            "Data" <- w179
          }
          frame #1 {
            n109 = Set Occurrence(w181) -> ()
          }
        }
        n110 = property on="Voltage Sequence" class="XYGraph (strict)"(error in=w166, "Active Plot"=w172, "Plot.Fill/Pt. Color"=u32 16777226) -> (error out=w153:errorcluster)  [unwired: 1 in, 1 out]
        n111 = call <userlib>:"BiasSpectroscopy SetTimings.vi"("Application ref in"=w154, "Initialization (NaN)"=w165, "End of Sweep (NaN)"=w164, "Error in (no error)"=w153) -> ("Application ref out"=w118:refnum<vi>, "Error out"=w115:errorcluster)  [unwired: 10 in]
        n112 = call <userlib>:"BiasSpectroscopy SetAdvancedProperties.vi"("Application ref in"=w118, "Reset Bias (no change)"=w114, "Z-Controller hold (no change)"=w114, "Error in (no error)"=w115) -> ("Application ref out"=w117:refnum<vi>, "Error out"=w116:errorcluster)  [unwired: 10 in]
        n113 = call <userlib>:"Voltage Set.vi"("Error in (no error)"=w116, "Bias (V)"=w155, "Application ref in"=w117) -> ("Error out"=w142:errorcluster, "Application ref out"=w146:refnum<vi>)  [unwired: 7 in]
        n114 = call <userlib>:"Ms to Wait with error cluster.vi"("error in (no error)"=w142, "milliseconds to wait"=u32 100) -> ("error out"=w141:errorcluster)  [unwired: 4 in, 1 out]
        n115 = call <userlib>:"Ctrl-on_off Set.vi"("error in (no error)"=w141, "Z Controller ON/OFF"=w160, "Application ref in"=w146) -> ("Application ref out"=w145:refnum<vi>)  [unwired: 7 in, 1 out]
      }
      frame True {
        n116 = local read "AllQuit"() -> (w212:bool)
      }
    }
  }
